vi "PH_gentec_P-Link.set SSE.vi"(0 "i ref in":refnum<vi>, 2 "VISA resource in":refnum<visa-resource-name>, 5 "error in":errorcluster) -> (11 "Timeout":bool, 13 "Data read":string[](array[string]), 14 "i ref out":refnum<vi>, 16 "VISA resource out":refnum<visa-resource-name>, 17 "Error":bool, 18 "Failure":bool, 19 "error out":errorcluster)   [LabVIEW 2014, in "PH_gentec_P-Link.lvlib"]
doc: "This VI writes wanted Settings to the Device and checks the result."
uses:
  PH_gentec_P-Link.lvlib
  instr.lib/Gentec-M-Link/gentec-M-Link - Driver.lvlib
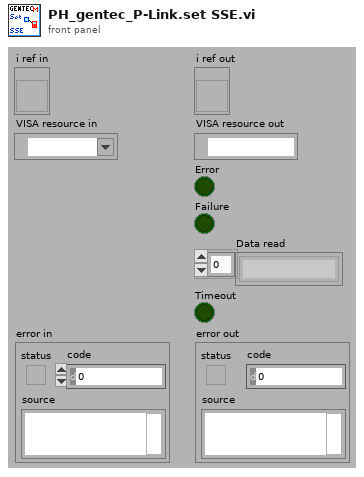
[diagram p1: front panel]
types:
  T1 = typedef "PH_gentec_P-Link.lvlib/PH_gentec_P-Link.i attribute.ctl" = cluster{"GUI References":cluster{"Wanted Head Settings":refnum<vi>, "Current Head Settings":refnum<vi>, "Set Auto Range":refnum<vi>, "Trigger Polarity":refnum<vi>, "Trigger Source":refnum<vi>, "Waveform Averages":refnum<vi>, "Continuous":refnum<vi>, "get one Value":refnum<vi>}, "Wanted Head Settings":T2, "Current Head Settings":T2}
  T2 = typedef "PH_gentec_P-Link.lvlib/PH_gentec_P-Link.Head Settings.ctl" = cluster{"Measurement Mode":T3, "Enable Anticipation":bool, "Set Auto Range":bool, "Block Signal":bool, "Set Head Attenuator":bool, "Enable SSE":bool, "Trigger Polarity":T4, "Trigger Source":T5, "Waveform Averages":T6, "Set Zero":i32, "Current Measurement":i32, "Start Data Flow":bool}
  T3 = typedef "gentec-M-Link - Driver.lvlib/gentec-M-Link.Measurement Mode.ctl" = u16
  T4 = typedef "gentec-M-Link - Driver.lvlib/gentec-M-Link.Trigger Polarity.ctl" = u16
  T5 = typedef "gentec-M-Link - Driver.lvlib/gentec-M-Link.Trigger Source.ctl" = u16
  T6 = typedef "gentec-M-Link - Driver.lvlib/gentec-M-Link.Waveform Averages.ctl" = u16
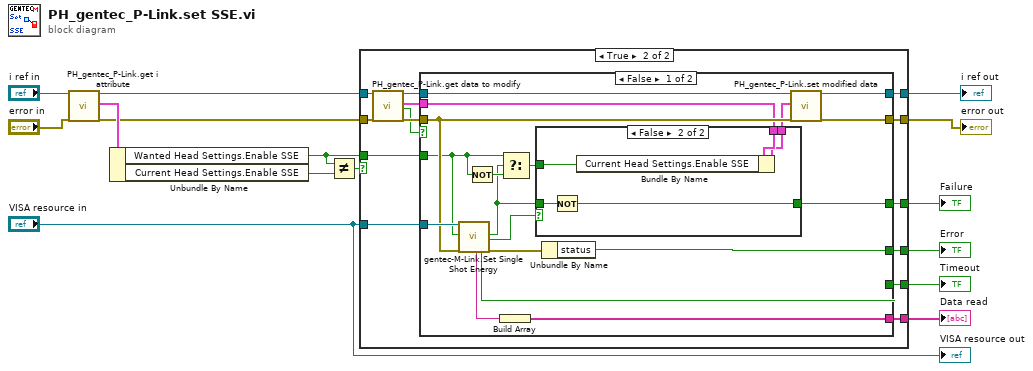
[diagram p0: block diagram]
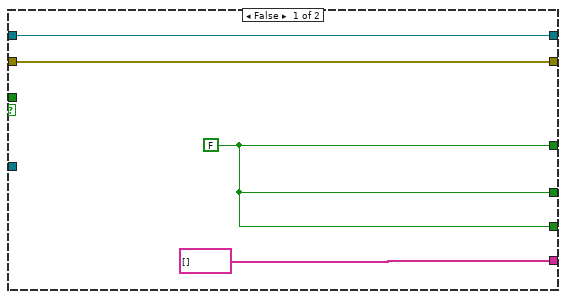
[diagram p2: hidden frame]
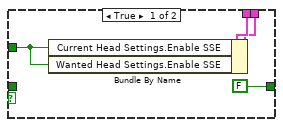
[diagram p3: hidden frame]
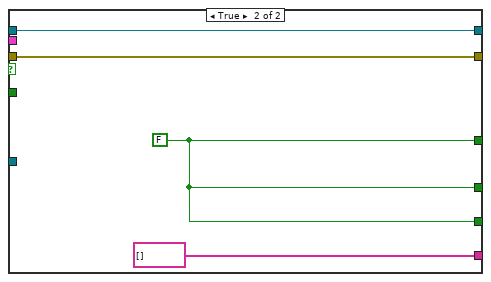
[diagram p4: hidden frame]
diagram:
  n1 = call "PH_gentec_P-Link.get i attribute.vi"("i ref in"="i ref in", "error in (no error)"="error in") -> ("i ref out"=w8:refnum<vi>, "i attribute"=w11:T1, "error out"=w10:errorcluster)  [unwired: 15 in]
  n2 = Unbundle By Name(w11) -> ("Wanted Head Settings.Enable SSE"=w13:bool, "Current Head Settings.Enable SSE"=w12:bool)
  n3 = Not Equal?(x=w13, y=w12) -> (x != y?=w1:bool)
  n4 = case shown="True" w1 {
    tunnel: [w16 w33] -> w15
    tunnel: [w17 w32] -> w14
    tunnel: w13 -> [_ w31]
    tunnel: w10 -> [w16 w26]
    tunnel: w8 -> [w17 w25]
    tunnel: "VISA resource in" -> [_ w24]
    tunnel: [w19 w23] -> w5
    tunnel: [w19 w22] -> w4
    tunnel: [w19 w21] -> w3
    tunnel: [string[] [] w20] -> w2
    frame False {
      w19 = FALSE
    }
    frame True {
      n5 = call "PH_gentec_P-Link.get data to modify.vi"("i ref in"=w25, "error in (no error)"=w26) -> ("i ref out"=w29:refnum<vi>, "i attribute"=w28:T1, "timed out"=w27:bool, "error out"=w30:errorcluster)  [unwired: 14 in]
      n6 = case shown="False" w27 {
        tunnel: w24 -> [w50 _]
        tunnel: [w46 w64] -> w32
        tunnel: [w45 w63] -> w33
        tunnel: w30 -> [w49 w63]
        tunnel: w29 -> [w51 w64]
        tunnel: w28 -> [w48 _]
        tunnel: w31 -> [w47 _]
        tunnel: [w43 w62] -> w23
        tunnel: [w42 w62] -> w22
        tunnel: [w41 w62] -> w21
        tunnel: [w40 string[] []] -> w20
        frame False {
          n7 = call "gentec-M-Link.Set Single Shot Energy.vi"("VISA resource In"=w50, "Enable Single Shot Energy"=w47, "error in (no error)"=w49) -> ("Data Read"=w34:string, "Read Timeout"=w41:bool, "Success"=w35:bool, "no Thermopyle Head"=w36:bool, "error out"=w39:errorcluster)  [unwired: 11 in, 1 out]
          n8 = Not(x=w47) -> (.not. x?=w38:bool)
          n9 = Build Array(w34) -> (w40:string[])
          n10 = Select(t=w47, s=w35, f=w38) -> (s? t:f=w37:bool)
          n11 = case shown="False" w36 {
            tunnel: w48 -> [w55 w60]
            tunnel: [w54 w59] -> w44
            tunnel: w37 -> [w53 w58]
            tunnel: w35 -> [_ w57]
            tunnel: [FALSE w56] -> w42
            frame True {
              n12 = Bundle By Name(cluster=w55, "Current Head Settings.Enable SSE"=w53, "Wanted Head Settings.Enable SSE"=w53) -> (w54:T1)
            }
            frame False {
              n13 = Not(x=w57) -> (.not. x?=w56:bool)
              n14 = Bundle By Name(cluster=w60, "Current Head Settings.Enable SSE"=w58) -> (w59:T1)
            }
          }
          n15 = Unbundle By Name(w39) -> ("status"=w43:bool)
          n16 = call "PH_gentec_P-Link.set modified data.vi"("i ref in"=w51, "i attribute"=w44, "error in (no error)"=w49) -> ("i ref out"=w46:refnum<vi>, "error out"=w45:errorcluster)  [unwired: 15 in]
        }
        frame True {
          w62 = FALSE
        }
      }
    }
  }
  "error out" <- w15
  "i ref out" <- w14
  "Error" <- w5
  "Failure" <- w4
  "Timeout" <- w3
  "Data read" <- w2
  "VISA resource out" <- "VISA resource in"
